vi "VNA_sweepPower.vi"(4 "Power Start (dbm)":dbl=-40.0, 7 "VNA Address":refnum<visa-resource-name>="GPIB0::15::INSTR", 11 "Transport":refnum<class "Transport.lvclass">=refnum) -> ()   [LabVIEW 2019]
uses:
  <userlib>/LevyLab/Transport/Transport/Transport.lvclass
  <userlib>/LevyLab/Transport/Control Experiment/Control Experiment.lvclass
  <userlib>/LevyLab/Lockin-Multichannel/Instrument.Lockin/Instrument.Lockin.lvclass
  <userlib>/LevyLab/Instrument Framework/subsystems/API/API.lvclass
  <userlib>/LevyLab/Configuration/Configuration.lvclass
  <userlib>/LevyLab/Instrument Framework/subsystems/HAL/HAL.lvclass
  <userlib>/LevyLab/Logger.PGSQL/Logger.PGSQL/Logger.PGSQL.lvclass
  <userlib>/LevyLab/Logger.Error/Logger.Error/Logger.Error.lvclass
  <userlib>/LevyLab/RemoteControl.ZMQ/RemoteControl.ZMQ/RemoteControl.ZMQ.lvclass
  <vilib>/addons/zeromq/zmq_socket.lvclass
  <userlib>/LevyLab/Lockin-Multichannel/Instrument.DAQ/Instrument.DAQ.lvclass
  <userlib>/LevyLab/Krohn Hite 7008/Inst.Krohn-Hite-7008/Inst.Krohn-Hite-7008.lvclass
  <userlib>/LevyLab/RemoteControl/RemoteControl/RemoteControl.lvclass
  <userlib>/LevyLab/Leiden API/Inst.TC.MNK/Inst.TC.MNK.lvclass
  <userlib>/LevyLab/Leiden API/FP-TC-Shared/FP-TC-Shared.lvclass
  <userlib>/LevyLab/Oxford-1820/Instrument.Oxford1820/Instrument.Oxford1820.lvclass
  <userlib>/LevyLab/Instrument Framework/Instrument Types/Cryostat/Instrument.Cryostat.lvclass
  <userlib>/LevyLab/Instrument Framework/Instrument Types/CBridge/Instrument.CBridge.lvclass
  <userlib>/LevyLab/Instrument Framework/Instrument Types/Delay Line/Instrument.DelayLine.lvclass
  <userlib>/LevyLab/Instrument Framework/Instrument Types/Strain/Instrument.Strain.lvclass
  <userlib>/LevyLab/Instrument Framework/Instrument Types/VNA/Instrument.VNA.lvclass
  <userlib>/LevyLab/Instrument Framework/Instrument Types/VSource/Instrument.VSource.lvclass
  <userlib>/LevyLab/Transport/Transport/Transport.lvclass/Transport.ctl
  <userlib>/LevyLab/Transport/Control Experiment/Control Experiment.lvclass/Control Experiment.ctl
  <instrlib>/Agilent 87XX Series/Agilent 87XX Series.lvlib
panel:
  in  "Experiment Folder":string="21-Psweep_132V"
  in  "Experiment Description":string="Power: -40 dbm to -20 dbm, 0.1 dbm step\nB=-1mT (true zero)\nT<30mK\nVbg(AO4) = 132.2 V\nPpump = -100 dBm\nfpump = 100MHz\n\nVd: 1.3V\nId: 9.55mA \nBW = 300 Hz \nAvg =1\n630MHz to 645MHz"
  in  "Power Step (dbm)":dbl=0.1
  in  "Power End (dbm)":dbl=-20.0
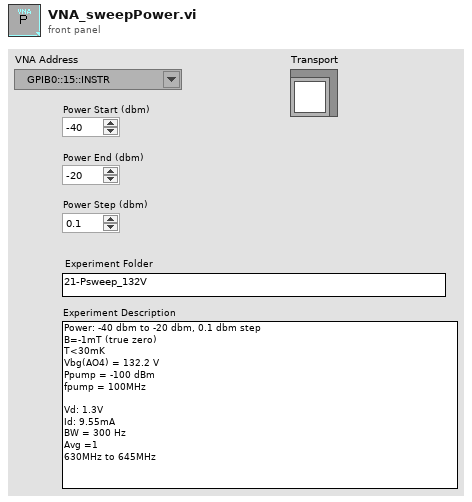
[diagram p1: front panel]
types:
  T1 = enum32{"Bad", "Idle", "Run top level", "Running"}
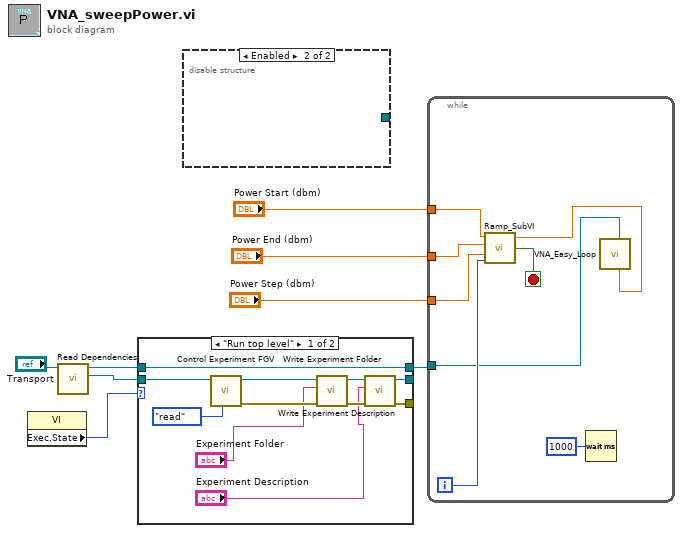
[diagram p0: block diagram]
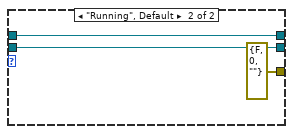
[diagram p2: hidden frame]
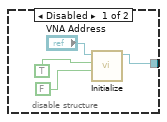
[diagram p3: hidden frame]
diagram:
  n1 = property class="VI"() -> ("Exec.State"=w5:T1)  [unwired: 2 in, 2 out]
  n2 = call <userlib>:"Read Dependencies.vi"("Transport"="Transport") -> ("C.E."=w4:refnum<class "Control Experiment.lvclass">, "Transport"=w3:refnum<class "Transport.lvclass">)  [unwired: 8 in, 1 out]
  n3 = case shown="\"Run top level\"" w5 {
    tunnel: [w15 errorcluster {"status"=FALSE, "code"=0, "source"=""} ("error out")] -> _
    tunnel: [w14 w22] -> _
    tunnel: w4 -> [w9 w22]
    tunnel: w3 -> [w10 w20]
    tunnel: [w10 w20] -> w1
    frame "Run top level" {
      n4 = call <userlib>:"Control Experiment FGV.vi"("Function"=enum16{"read", "write"}."read", "Control Experiment.lvclass"=w9) -> ("error out"=w18:errorcluster, "Control Experiment.lvclass out"=w19:refnum<class "Control Experiment.lvclass">)  [unwired: 8 in]
      n5 = call <userlib>:"Write Experiment Folder.vi"("error in (no error)"=w18, "Experiment Folder"="Experiment Folder", "Control Experiment in"=w19) -> ("error out"=w16:errorcluster, "Control Experiment out"=w17:refnum<class "Control Experiment.lvclass">)  [unwired: 7 in]
      n6 = call <userlib>:"Write Experiment Description.vi"("error in (no error)"=w16, "Experiment Description"="Experiment Description", "Control Experiment in"=w17) -> ("error out"=w15:errorcluster, "Control Experiment out"=w14:refnum<class "Control Experiment.lvclass">)  [unwired: 7 in]
    }
    frame "Running", Default {
    }
  }
  n7 = disable-structure shown="Enabled" {
    disable-tunnel: [w23 _] -> _
    frame Disabled {
      n8 = call <instrlib>:"Initialize.vi"("reset"=FALSE, "ID query"=TRUE, "VISA resource name"="VNA Address") -> ("VISA resource name out"=w23:refnum<visa-resource-name>)  [unwired: 7 in, 1 out]
    }
    frame Enabled {
    }
  }
  n9 = while {
    tunnel: "Power Start (dbm)" -> [w34]
    tunnel: "Power End (dbm)" -> [w33]
    tunnel: "Power Step (dbm)" -> [w32]
    tunnel: w1 -> [w27]
    i -> [w31]
    stop <- w30 stop-if-true
    n10 = call <userlib>:"Ramp_SubVI.vi"("index"=w31, "step"=w32, "end"=w33, "start"=w34) -> ("Stop?"=w30:bool, "Numeric"=w29:dbl)  [unwired: 1 in]
    n11 = Wait (ms)(milliseconds to wait=u32 1000) -> ()  [unwired: 1 out]
    n12 = call "VNA_Easy_Loop.vi"("Power (dbm)"=w29, "Transport"=w27) -> ()  [unwired: 8 in, 2 out]
  }
